vi "LDA+_An_Analysis_mode.vi"(6 "Second Graph":T2={"Plot 1"=1, "Plot 2"=2, "Save graph"=0, "Plot Type"=enum."Voltage trace"} {"Save graph" items=["Do not save plot", "Save plot"]; "Plot 2" items=["Nothing", "Prop 2 (U)"]; "Plot 1" items=["Nothing", "Prop 2 (U)"]}, 9 "First Graph":T2={"Plot 1"=1, "Plot 2"=2, "Save graph"=0, "Plot Type"=enum."Voltage trace"} {"Save graph" items=["Do not save plot", "Save plot"]; "Plot 2" items=["Nothing", "Prop 2 (U)"]; "Plot 1" items=["Nothing", "Prop 2 (U)"]}) -> (0 "Second Graph out":T2={"Plot 1"=1, "Plot 2"=2, "Save graph"=0, "Plot Type"=enum."Voltage trace"} {"Save graph" items=["Do not save plot", "Save plot"]; "Plot 2" items=["Nothing", "Prop 2 (U)"]; "Plot 1" items=["Nothing", "Prop 2 (U)"]}, 3 "First Graph out":T2={"Plot 1"=1, "Plot 2"=2, "Save graph"=0, "Plot Type"=enum."Voltage trace"} {"Save graph" items=["Do not save plot", "Save plot"]; "Plot 2" items=["Nothing", "Prop 2 (U)"]; "Plot 1" items=["Nothing", "Prop 2 (U)"]})   [LabVIEW 2011]
uses:
  Controls/Graph_Type.ctl
  Globals/Meas_global.vi
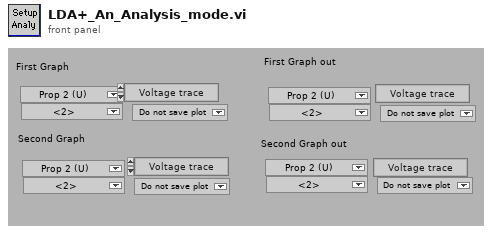
[diagram p1: front panel]
types:
  T1 = typedef "Graph_Type.ctl" = enum16{"Show no graph", "Voltage trace", "Velocity trace", "Vel histogram", "Spectrum", "f.E(f) v Log f", "Auto-Corr"}
  T2 = cluster{"Plot 1":u16, "Plot 2":u16, "Save graph":u16, "Plot Type":T1}
  T3 = typedef "Analysis_info_cluster.ctl" = cluster{"Colour":u32, "Inst type":T4, "Inst name":string, "Symbol":string, "Code name":string, "Extra Info":string, "Inst Array":T5, "Index":i32, "Voltage Index":i32, "Extra Titles":string[], "Extra Values":string[], "Eng Values":dbl[], "Time (ms)":dbl[], "TT / Voltage":dbl[], "U":dbl, "u^2":dbl, "u^3":dbl, "u^4":dbl, "Skew_u":dbl, "Kurt_u":dbl, "Sd Error in Mean":dbl, "% u'/U":dbl, "X":dbl, "Y":dbl, "Z":dbl, "Spectra":T6, "Autocorrelation":T6, "Timescale integral to 25%":dbl, "Sd Error in Variance":dbl, "Calib File":path, "Calib Constants":dbl[], "Histogram":T6, "Output Position":bool, "Full Stats":bool}
  T4 = typedef "Inst_type.ctl" = enum16{"Propeller anemometer", "Raw voltage", "Pressure Transducer", "Pitot-static tube", "Preston tube", "Hot wire", "Cross wire 1", "Cross wire 2", "Generic Linear", "Generic Polynomial", "Generic BackPoly", "Fast FID", "Thermocouple", "Cold wire", "Pulsed Wire", "LDA Vel", "LDA Tran time", "LDA Arr time"}
  T5 = typedef "Instrument_Array.ctl" = enum16{"PWA", "LDA", "Analogue"}
  T6 = typedef "XY_Plot_Cluster.ctl" = cluster{"First Name":string, "Second Name":string, "X axis name":string, "Y axis name":string, "X array":dbl[], "Y array":dbl[]}
  T7 = enum16{"Show no graph", "Voltage trace", "Velocity trace", " Vel histogram", "Spectrum", "f.E(f) v Log f", "Auto-Corr"}
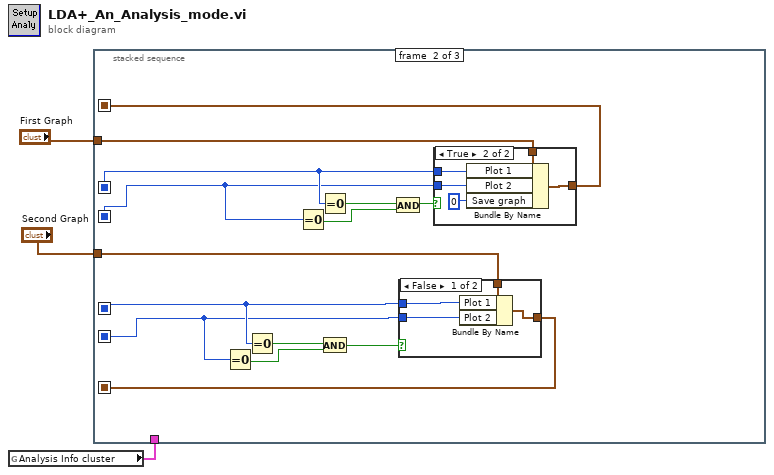
[diagram p0: block diagram]
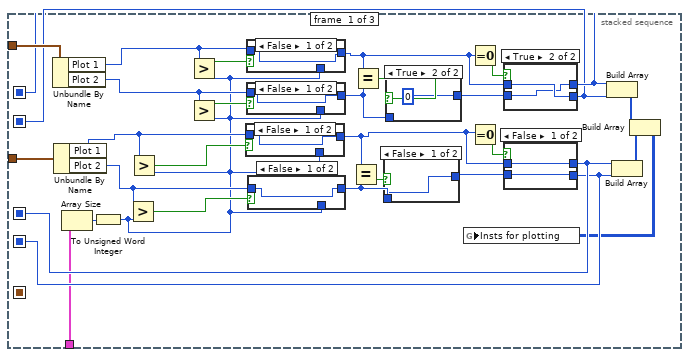
[diagram p2: hidden frame]
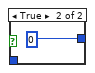
[diagram p10: hidden frame]
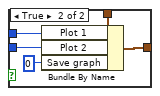
[diagram p11: hidden frame]
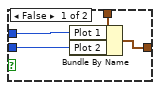
[diagram p12: hidden frame]
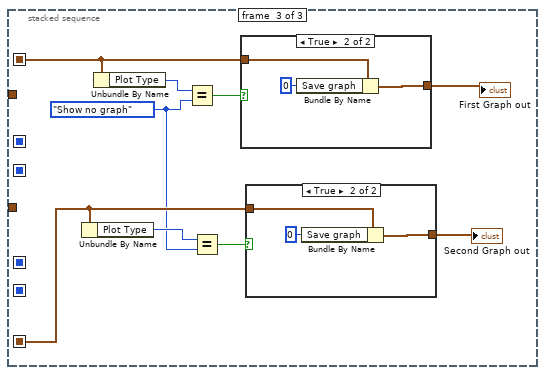
[diagram p13: hidden frame]
diagram:
  n1 = global read "Meas_global.vi" "Analysis Info cluster"() -> (w1:T3[])
  n2 = stacked-sequence {
    seq-local: [w15 _ _] -> [_ w64 _]
    seq-local: [w14 _ _] -> [_ w63 _]
    seq-local: [w10 _ _] -> [_ w58 _]
    seq-local: [w9 _ _] -> [_ w57 _]
    seq-local: [_ w54 _] -> [_ _ w92]
    seq-local: [_ w55 _] -> [_ _ w88]
    tunnel: "First Graph" -> [w24 w67 _]
    tunnel: "Second Graph" -> [w23 w61 _]
    tunnel: w1 -> [w4 _ _]
    frame #0 {
      n3 = Unbundle By Name(w24) -> ("Plot 1"=w22:u16, "Plot 2"=w21:u16)
      n4 = Unbundle By Name(w23) -> ("Plot 1"=w20:u16, "Plot 2"=w19:u16)
      n5 = Array Size(array=w4) -> (size(s)=w33:i32)
      n6 = To Unsigned Word Integer(number=w33) -> (unsigned 16bit integer=w5:u16)
      n7 = Greater?(x=w19, y=w5) -> (0:w29:bool)
      n8 = Greater?(x=w20, y=w5) -> (0:w28:bool)
      n9 = Greater?(x=w22, y=w5) -> (0:w26:bool)
      n10 = Greater?(x=w21, y=w5) -> (0:w27:bool)
      n11 = case shown="False" w28 {
        tunnel: [w48 w49] -> w12
        tunnel: w20 -> [w48 _]
        tunnel: w5 -> [_ w49]
        frame False {
        }
        frame True {
        }
      }
      n12 = case shown="False" w26 {
        tunnel: [w44 w45] -> w17
        tunnel: w22 -> [w44 _]
        tunnel: w5 -> [_ w45]
        frame False {
        }
        frame True {
        }
      }
      n13 = case shown="False" w27 {
        tunnel: [w46 w47] -> w30
        tunnel: w21 -> [w46 _]
        tunnel: w5 -> [_ w47]
        frame False {
        }
        frame True {
        }
      }
      n14 = case shown="False" w29 {
        tunnel: [w50 w51] -> w32
        tunnel: w19 -> [w50 _]
        tunnel: w5 -> [_ w51]
        frame False {
        }
        frame True {
        }
      }
      n15 = Equal?(x=w12, y=w32) -> (x = y?=w31:bool)
      n16 = Equal?(x=w17, y=w30) -> (x = y?=w25:bool)
      n17 = case shown="False" w31 {
        tunnel: [w52 u16 0] -> w11
        tunnel: w32 -> [w52 _]
        frame False {
        }
        frame True {
        }
      }
      n18 = case shown="True" w25 {
        tunnel: [w42 u16 0] -> w16
        tunnel: w30 -> [w42 _]
        frame False {
        }
        frame True {
        }
      }
      n19 = Equal To 0?(x=w17) -> (x = 0?=w18:bool)
      n20 = Equal To 0?(x=w12) -> (x = 0?=w13:bool)
      n21 = case shown="True" w18 {
        tunnel: [w38 w41] -> w14
        tunnel: w17 -> [w39 w41]
        tunnel: [w39 w40] -> w15
        tunnel: w16 -> [w38 w40]
        frame False {
        }
        frame True {
        }
      }
      n22 = case shown="False" w13 {
        tunnel: [w34 w37] -> w9
        tunnel: w12 -> [w35 w37]
        tunnel: [w35 w36] -> w10
        tunnel: w11 -> [w34 w36]
        frame False {
        }
        frame True {
        }
      }
      n23 = Build Array(w15, w14) -> (w8:u16[])
      n24 = Build Array(w10, w9) -> (w7:u16[])
      n25 = Build Array(w8, w7) -> (w6:u16[][])
      n26 = global write "Meas_global.vi" "Insts for plotting"(w6) -> ()
    }
    frame #1 {
      n27 = Equal To 0?(x=w57) -> (x = 0?=w60:bool)
      n28 = Equal To 0?(x=w58) -> (x = 0?=w59:bool)
      n29 = Equal To 0?(x=w63) -> (x = 0?=w65:bool)
      n30 = Equal To 0?(x=w64) -> (x = 0?=w66:bool)
      n31 = And(x=w59, y=w60) -> (x .and. y?=w56:bool)
      n32 = And(x=w66, y=w65) -> (x .and. y?=w62:bool)
      n33 = case shown="False" w56 {
        tunnel: [w71 w76] -> w55
        tunnel: w57 -> [w70 w75]
        tunnel: w58 -> [w69 w74]
        tunnel: w61 -> [w68 w73]
        frame False {
          n34 = Bundle By Name(cluster=w68, "Plot 1"=w69, "Plot 2"=w70) -> (w71:T2)
        }
        frame True {
          n35 = Bundle By Name(cluster=w73, "Plot 1"=w74, "Plot 2"=w75, "Save graph"=0) -> (w76:T2)
        }
      }
      n36 = case shown="True" w62 {
        tunnel: [w80 w85] -> w54
        tunnel: w63 -> [w79 w84]
        tunnel: w64 -> [w78 w83]
        tunnel: w67 -> [w77 w82]
        frame False {
          n37 = Bundle By Name(cluster=w77, "Plot 1"=w78, "Plot 2"=w79) -> (w80:T2)
        }
        frame True {
          n38 = Bundle By Name(cluster=w82, "Plot 1"=w83, "Plot 2"=w84, "Save graph"=0) -> (w85:T2)
        }
      }
    }
    frame #2 {
      w87 = T7."Show no graph" ("Plot Type")
      n39 = Unbundle By Name(w88) -> ("Plot Type"=w89:T1)
      n40 = Unbundle By Name(w92) -> ("Plot Type"=w94:T1)
      n41 = Equal?(x=w94, y=w87) -> (x = y?=w93:bool)
      n42 = Equal?(x=w89, y=w87) -> (x = y?=w90:bool)
      n43 = case shown="True" w93 {
        tunnel: w92 -> [w99 w102]
        tunnel: [w99 w100] -> w91
        frame False {
        }
        frame True {
          n44 = Bundle By Name(cluster=w102, "Save graph"=u16 0) -> (w100:T2)
        }
      }
      "First Graph out" <- w91
      n45 = case shown="True" w90 {
        tunnel: w88 -> [w95 w98]
        tunnel: [w95 w96] -> w86
        frame False {
        }
        frame True {
          n46 = Bundle By Name(cluster=w98, "Save graph"=u16 0) -> (w96:T2)
        }
      }
      "Second Graph out" <- w86
    }
  }
